vi "CSClassUtilities.CopyAndRenameClass.vi"() -> (8 "Done?":bool)   [LabVIEW 2014]
doc: "This tool makes a copy of a class, it chanches only the classname and all called sub-vi´s inside the vi-hierachie\n\nIt does only support CS-3.10 classes (no private, protected,public Folder) !\nIt doesnt copy the Inheritance-Folder !\nIt does not sort the library, it only generates it !\n\nIf ou want to have support for one of these, feel free to modify this tool !!\n\nAlexander Schwinn (al.schwinn@gsi.de)"
uses:
  CSClass/CS_Core/CSSystem/CSSystemLib/CSSystemLib.lvlib
panel:
  in  "Boolean":bool
  out "Tab control":T1(tab)
  in  "Continue1":bool
  in  "...or type in the classname here":string
  in  "Select the class you want to copy & rename":i32(listbox)
  in  "Continue2":bool
  in  "New Folder for the copy":path
  in  "use the folder of the old class":bool=TRUE
  in  "choose a classname for the copy":string
  in  "Continue3":bool
  # "This tool generates a copy of an existing class, and gives a new name to this copy. You can use it to build new classes, or simply to rename an existing class.\n\n1) This tool  will open and rename a couple of VIs. It is strongly recommended to use this tool not from a project but directly after launching LabVIEW!\n\n2) This tool will only work on classes that are below the \".../CSClass\" folder.\n\n3) This tool only works on CS v3.10 and higher classes\n       -  it doesnt copy the Inheritance-folder !\n       -  it does not sort the library, it only generates it ! \n       -  feel free to modify this tool, to add some functionality !!"
  # "1) LabVIEW  now copies and renames all necessery files.\n\n2) When done, it is recommended to exit and restart LabVIEW.\n\n3) If you have created a new class, it is a good idea to modify the icons of\n     the methods of this class. An easy way to do that, is the usage of the\n     \"CSClassUtilities.dublicate icon tool.vi\" ."
  # "Designer:   Alexander Schwinn (al.schwinn@gsi.de)"
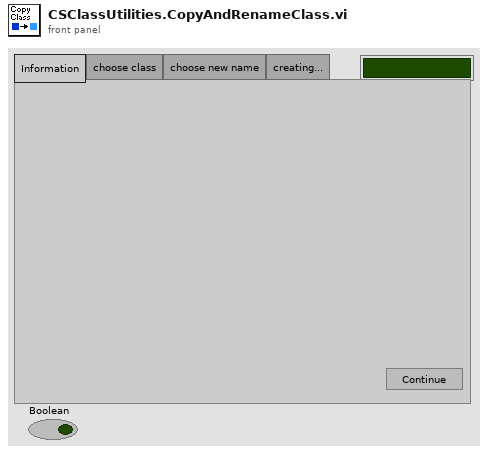
[diagram p1: front panel]
types:
  T1 = enum32{"Information", "choose class", "choose new name", "creating..."}
  T2 = enum32{"invalid scope", "public", "private", "protected"}
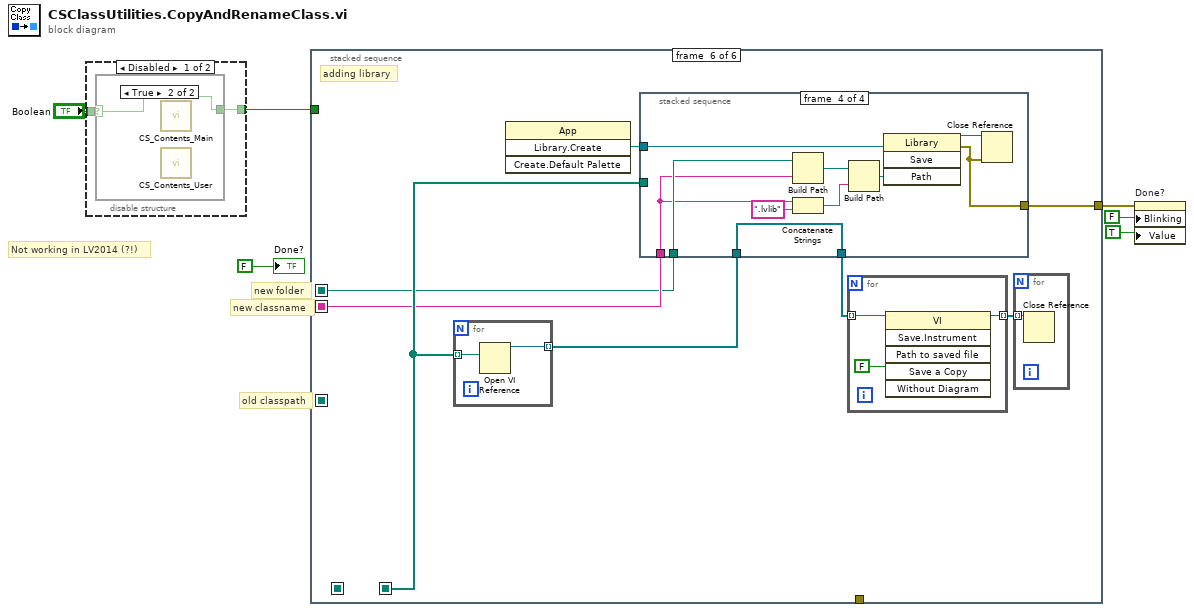
[diagram p0: block diagram]
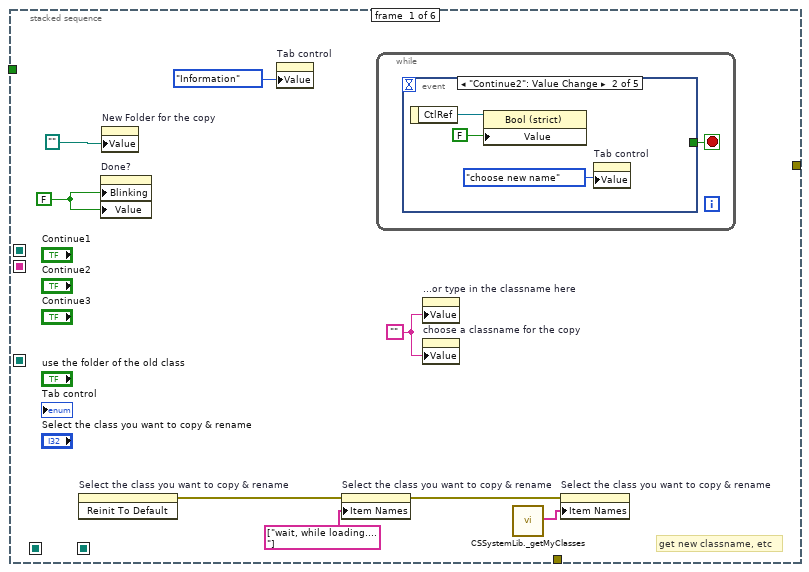
[diagram p4: hidden frame]
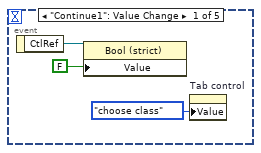
[diagram p5: hidden frame]
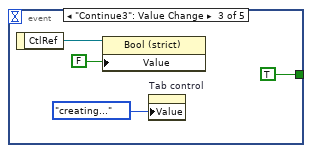
[diagram p6: hidden frame]
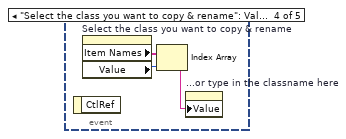
[diagram p7: hidden frame]
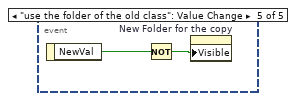
[diagram p8: hidden frame]
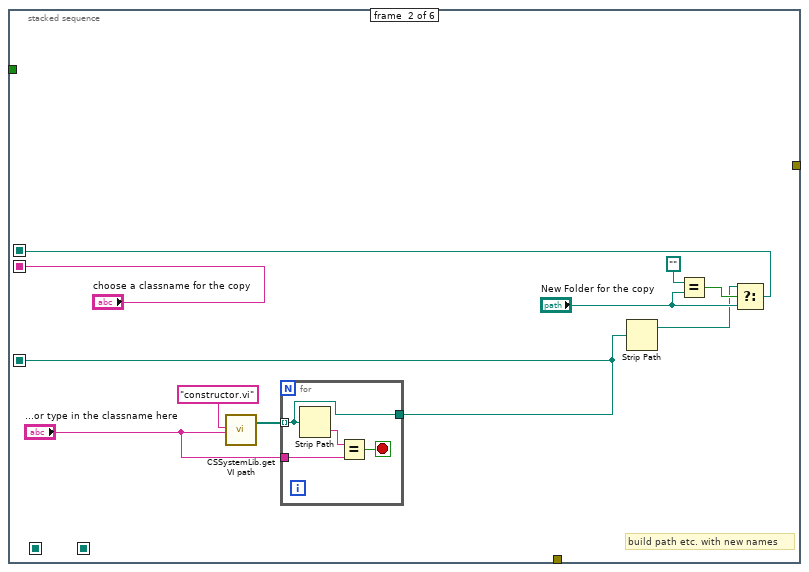
[diagram p9: hidden frame]
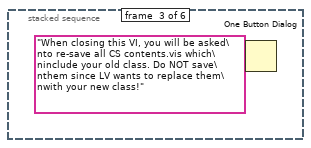
[diagram p10: hidden frame]
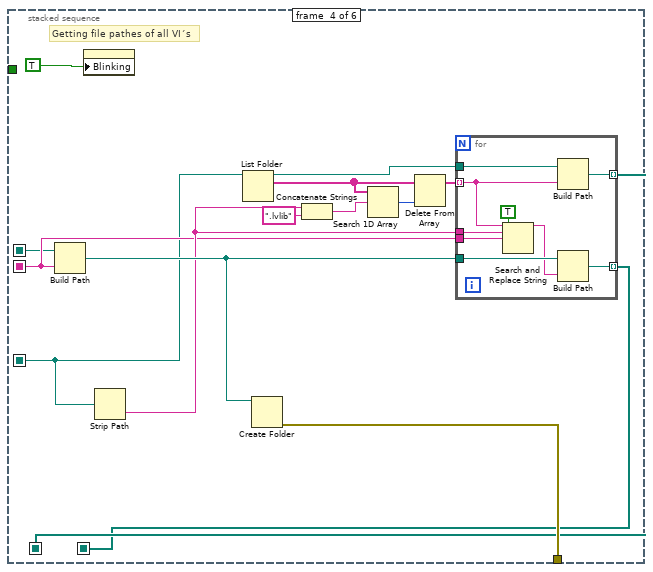
[diagram p11: hidden frame]
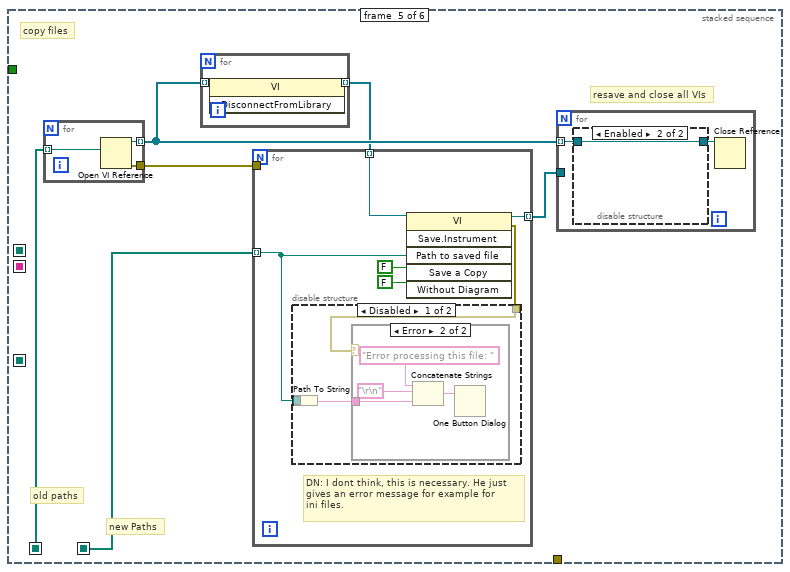
[diagram p12: hidden frame]
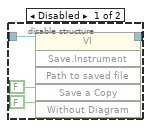
[diagram p13: hidden frame]
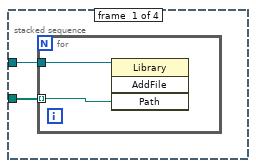
[diagram p16: hidden frame]
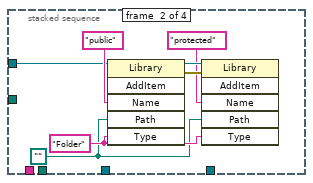
[diagram p17: hidden frame]
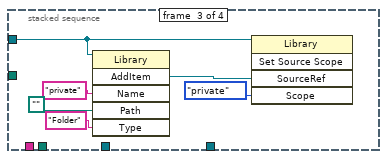
[diagram p18: hidden frame]
diagram:
  # "Not working in LV2014 (?!)"
  # "old classpath"
  # "new folder"
  # "new classname"
  n1 = disable-structure shown="Disabled" {
    disable-tunnel: "Boolean" -> [w8 _]
    disable-tunnel: [w7 _] -> w1
    frame Disabled {
      n2 = case shown="True" w8 {
        selector: w8 -> [_ w9]
        tunnel: [_ w9] -> w7
        frame False {
        }
        frame True {
          n3 = call "CS_Contents_Main.vi"() -> ()  [unwired: 1 in]
          n4 = call "CS_Contents_User.vi"() -> ()  [unwired: 1 in]
        }
      }
    }
    frame Enabled {
    }
  }
  n5 = stacked-sequence {
    seq-local: [_ _ _ w61 _ _] -> [_ _ _ _ w77 _]
    seq-local: [_ _ _ w60 _ _] -> [_ _ _ _ w75 w110]
    seq-local: [_ "choose a classname for the copy" _ _ _ _] -> [_ _ _ w52 _ w105]
    seq-local: [_ w38 _ _ _ _] -> [_ _ _ w50 _ w104]
    seq-local: [_ w34 _ _ _ _] -> [_ _ _ w51 _ _]
    tunnel: [_ _ _ _ _ w106] -> w4
    tunnel: [_ _ _ w62 _ _] -> _
    tunnel: w1 -> [_ _ _ _ _ _]
    frame #0 {
      w12 = ""
      w11 = FALSE ("Done?")
      # "get new classname, etc"
      n6 = invoke on="Select the class you want to copy & rename" class="LstBox (strict)" method="Reinit To Default"() -> (error out=w10:errorcluster)  [unwired: 3 in, 2 out]
      n7 = property on="Done?" class="Bool (strict)"("Blinking"=w11, "Value"=w11) -> ()  [unwired: 2 in, 2 out]
      n8 = property on="New Folder for the copy" class="Path"("Value"=path "") -> ()  [unwired: 2 in, 2 out]
      n9 = property on="Tab control" class="TabCtl (strict)"("Value"=T1."Information" ("Tab control")) -> ()  [unwired: 2 in, 2 out]
      n10 = property on="Select the class you want to copy & rename" class="LstBox (strict)"(error in=w10, "Item Names"=string[] ["wait, while loading...."]) -> (error out=w16:errorcluster)  [unwired: 1 in, 1 out]
      n11 = while {
        stop <- w18 stop-if-true
        n12 = event shown="[1] \"Continue2\": Value Change" {
          selector: _ -> [_ _ _ _ _]
          dyn-events: _ -> [_ _ _ _ _]
          timeout: _ -> [_ _ _ _ _]
          tunnel: [_ _ TRUE _ _] -> w18
          event "Continue1": Value Change {
            n13 = event-data() -> ("CtlRef"=w19:refnum<vi>)  [unwired: 1 in]
            n14 = property class="Bool (strict)"(reference=w19, "Value"=FALSE) -> ()  [unwired: 1 in, 2 out]
            n15 = property on="Tab control" class="TabCtl (strict)"("Value"=T1."choose class" ("Tab control")) -> ()  [unwired: 2 in, 2 out]
          }
          event "Continue2": Value Change {
            n16 = event-data() -> ("CtlRef"=w23:refnum<vi>)  [unwired: 1 in]
            n17 = property class="Bool (strict)"(reference=w23, "Value"=FALSE) -> ()  [unwired: 1 in, 2 out]
            n18 = property on="Tab control" class="TabCtl (strict)"("Value"=T1."choose new name" ("Tab control")) -> ()  [unwired: 2 in, 2 out]
          }
          event "Continue3": Value Change {
            n19 = event-data() -> ("CtlRef"=w27:refnum<vi>)  [unwired: 1 in]
            n20 = property class="Bool (strict)"(reference=w27, "Value"=FALSE) -> ()  [unwired: 1 in, 2 out]
            n21 = property on="Tab control" class="TabCtl (strict)"("Value"=T1."creating..." ("Tab control")) -> ()  [unwired: 2 in, 2 out]
          }
          event "Select the class you want to copy & rename": Value Change {
            n22 = event-data() -> ()  [unwired: 1 in, 1 out]
            n23 = property on="Select the class you want to copy & rename" class="LstBox (strict)"() -> ("Item Names"=w31:string[], "Value"=w30:i32)  [unwired: 2 in, 2 out]
            n24 = Index Array(array=w31, index=w30) -> (element=w29:string)
            n25 = property on="...or type in the classname here" class="Str"("Value"=w29) -> ()  [unwired: 2 in, 2 out]
          }
          event "use the folder of the old class": Value Change {
            n26 = event-data() -> ("NewVal"=w33:bool)  [unwired: 1 in]
            n27 = Not(x=w33) -> (.not. x?=w32:bool)
            n28 = property on="New Folder for the copy" class="Path"("Visible"=w32) -> ()  [unwired: 2 in, 2 out]
          }
        }
      }
      n29 = property on="...or type in the classname here" class="Str"("Value"=w12) -> ()  [unwired: 2 in, 2 out]
      n30 = property on="choose a classname for the copy" class="Str"("Value"=w12) -> ()  [unwired: 2 in, 2 out]
      n31 = call "CSSystemLib._getMyClasses.vi"() -> ("myClasses"=w14:string[])  [unwired: 18 in, 1 out]
      n32 = property on="Select the class you want to copy & rename" class="LstBox (strict)"(error in=w16, "Item Names"=w14) -> ()  [unwired: 1 in, 2 out]
    }
    frame #1 {
      # "build path etc. with new names"
      n33 = call "CSSystemLib.get VI path.vi"("method"="constructor.vi" ("Method"), "class"="...or type in the classname here") -> ("Directories"=w35:path[])  [unwired: 15 in, 2 out]
      n34 = for {
        tunnel: "...or type in the classname here" -> [w46]
        tunnel: w35 -> [w44] mode=indexing
        tunnel: [w44] -> w34
        stop <- w45 stop-if-true
        n35 = Strip Path(path=w44) -> (name=w47:string)  [unwired: 1 out]
        n36 = Equal?(x=w47, y=w46) -> (x = y?=w45:bool)
      }
      n37 = Strip Path(path=w34) -> (stripped path=w37:path)  [unwired: 1 out]
      n38 = Equal?(x=path "", y="New Folder for the copy") -> (x = y?=w40:bool)
      n39 = Select(t=w37, s=w40, f="New Folder for the copy") -> (s? t:f=w38:path)
    }
    frame #2 {
      n40 = One Button Dialog(message="When closing this VI, you will be asked\nto re-save all CS contents.vis which\ninclude your old class. Do NOT save\nthem since LV wants to replace them\nwith your new class!") -> ()  [unwired: 1 in, 1 out]
    }
    frame #3 {
      # "Getting file pathes of all VI´s"
      n41 = Build Path(base path=w50, name or relative path=w52) -> (appended path=w63:path)
      n42 = property on="Done?" class="Bool (strict)"("Blinking"=TRUE) -> ()  [unwired: 2 in, 2 out]
      n43 = Strip Path(path=w51) -> (name=w53:string)  [unwired: 1 out]
      n44 = List Folder(path=w51) -> (path out=w59:path, filenames=w55:string[])  [unwired: 3 in, 2 out]
      n45 = Create Folder(path (use dialog)=w63) -> (error out=w62:errorcluster)  [unwired: 2 in, 2 out]
      n46 = Concatenate Strings(w53, ".lvlib" ("regular expression")) -> (w57:string)
      n47 = Search 1D Array(1D array=w55, element=w57) -> (index of element=w56:i32)  [unwired: 1 in]
      n48 = Delete From Array(array=w55, index=w56) -> (array with subset deleted=w54:string[])  [unwired: 1 in, 1 out]
      n49 = for {
        tunnel: w54 -> [w66] mode=indexing
        tunnel: w59 -> [w72]
        tunnel: [w71] -> w61 mode=indexing
        tunnel: w63 -> [w70]
        tunnel: w53 -> [w69]
        tunnel: w52 -> [w68]
        tunnel: [w67] -> w60 mode=indexing
        n50 = Search and Replace String(replace all?=TRUE ("replace all? (F)"), input string=w66, search string=w69, replace string=w68) -> (result string=w64:string)  [unwired: 4 in, 3 out]
        n51 = Build Path(base path=w72, name or relative path=w66) -> (appended path=w71:path)
        n52 = Build Path(base path=w70, name or relative path=w64) -> (appended path=w67:path)
      }
    }
    frame #4 {
      # "copy files"
      # "old paths"
      # "new Paths"
      # "resave and close all VIs"
      n53 = for {
        tunnel: w77 -> [w83] mode=indexing
        tunnel: [w82] -> w78
        tunnel: [w81] -> w74 mode=indexing
        n54 = Open VI Reference(vi path=w83) -> (vi reference=w81:refnum<vi>, error out=w82:errorcluster)  [unwired: 5 in]
      }
      n55 = for {
        tunnel: w74 -> [w80] mode=indexing
        tunnel: [w79] -> w73 mode=indexing
        n56 = invoke class="VI" method="DisconnectFromLibrary"(reference=w80) -> (reference out=w79:refnum<vi>)  [unwired: 2 in, 2 out]
      }
      n57 = for {
        tunnel: w78 -> [_]
        tunnel: [w96] -> w76 mode=indexing
        tunnel: w75 -> [w92] mode=indexing
        tunnel: w73 -> [w91] mode=indexing
        # "DN: I dont think, this is necessary. He just\ngives an error message for example for\nini files."
        n58 = invoke class="VI" method="Save.Instrument"(reference=w91, "Path to saved file"=w92, "Save a Copy"=FALSE, "Without Diagram"=FALSE) -> (reference out=w96:refnum<vi>, error out=w93:errorcluster)  [unwired: 2 in, 4 out]
        n59 = disable-structure shown="Disabled" {
          disable-tunnel: w93 -> [w99 _]
          disable-tunnel: w92 -> [w98 _]
          frame Disabled {
            n60 = Path To String(path=w98) -> (string=w97:string)
            n61 = case shown="Error" w99 {
              tunnel: w97 -> [_ w101]
              frame No Error {
              }
              frame Error {
                n62 = Concatenate Strings("Error processing this file: ", "\r\n", w101) -> (w103:string)
                n63 = One Button Dialog(message=w103) -> ()  [unwired: 1 in, 1 out]
              }
            }
          }
          frame Enabled {
          }
        }
      }
      n64 = for {
        tunnel: w74 -> [w84] mode=indexing
        tunnel: w76 -> [_]
        n65 = disable-structure shown="Enabled" {
          disable-tunnel: [w89 w90] -> w85
          disable-tunnel: w84 -> [w88 w90]
          frame Disabled {
            n66 = invoke class="VI" method="Save.Instrument"(reference=w88, "Save a Copy"=FALSE, "Without Diagram"=FALSE) -> (reference out=w89:refnum<vi>)  [unwired: 3 in, 5 out]
          }
          frame Enabled {
          }
        }
        n67 = Close Reference(reference=w85) -> ()  [unwired: 1 in, 1 out]
      }
    }
    frame #5 {
      # "adding library"
      n68 = for {
        tunnel: w110 -> [w144] mode=indexing
        tunnel: [w143] -> w109 mode=indexing
        n69 = Open VI Reference(vi path=w144) -> (vi reference=w143:refnum<vi>)  [unwired: 5 in, 1 out]
      }
      n70 = invoke class="App" method="Library.Create"() -> ("Create Library"=w107:refnum<vi>)  [unwired: 4 in, 3 out]
      n71 = stacked-sequence {
        tunnel: w110 -> [w113 _ _ _]
        tunnel: w109 -> [_ _ _ w133]
        tunnel: w104 -> [_ _ _ w132]
        tunnel: w105 -> [_ _ _ w130]
        tunnel: w107 -> [w112 w119 w123 w134]
        tunnel: [_ _ _ w133] -> w108
        tunnel: [_ _ _ w129] -> w106
        frame #0 {
          n72 = for {
            tunnel: w112 -> [w115]
            tunnel: w113 -> [w114] mode=indexing
            n73 = invoke class="Library" method="AddFile"(reference=w115, "Path"=w114) -> ()  [unwired: 2 in, 4 out]
          }
        }
        frame #1 {
          w117 = path ""
          w118 = "Folder" ("Type")
          n74 = invoke class="Library" method="AddItem"(reference=w119, "Name"="public", "Path"=w117, "Type"=w118) -> (reference out=w121:refnum<vi>, error out=w120:errorcluster)  [unwired: 2 in, 4 out]
          n75 = invoke class="Library" method="AddItem"(reference=w121, error in=w120, "Name"="protected", "Path"=w117, "Type"=w118) -> ()  [unwired: 1 in, 6 out]
        }
        frame #2 {
          n76 = invoke class="Library" method="AddItem"(reference=w123, "Name"="private", "Path"=path "", "Type"="Folder") -> ("AddItem"=w124:refnum<vi>)  [unwired: 2 in, 5 out]
          n77 = invoke class="Library" method="Set Source Scope"(reference=w123, "SourceRef"=w124, "Scope"=T2."private" ("scope")) -> ()  [unwired: 2 in, 5 out]
        }
        frame #3 {
          n78 = Build Path(base path=w132, name or relative path=w130) -> (appended path=w131:path)
          n79 = Concatenate Strings(w130, ".lvlib" ("string")) -> (w137:string)
          n80 = Build Path(base path=w131, name or relative path=w137) -> (appended path=w135:path)
          n81 = invoke class="Library" method="Save"(reference=w134, "Path"=w135) -> (reference out=w136:refnum<vi>, error out=w129:errorcluster)  [unwired: 2 in, 2 out]
          n82 = Close Reference(reference=w136, error in (no error)=w129) -> ()  [unwired: 1 out]
        }
      }
      n83 = for {
        tunnel: w108 -> [w142] mode=indexing
        tunnel: [w140] -> w111 mode=indexing
        n84 = invoke class="VI" method="Save.Instrument"(reference=w142, "Save a Copy"=FALSE) -> (reference out=w140:refnum<vi>)  [unwired: 4 in, 5 out]
      }
      n85 = for {
        tunnel: w111 -> [w139] mode=indexing
        n86 = Close Reference(reference=w139) -> ()  [unwired: 1 in, 1 out]
      }
    }
  }
  n87 = property on="Done?" class="Bool (strict)"(error in=w4, "Blinking"=FALSE, "Value"=TRUE ("Done?")) -> ()  [unwired: 1 in, 2 out]
  "Done?" <- FALSE ("Blinking")
